vi "[SubVI]PMC.vi"(4 "Weight":dbl format="%#_13g", 6 "Speed":dbl format="%#_13g", 7 "Right Stride":bool, 9 "Offset  array":sgl[](array[numeric]), 10 "Max torque in":sgl=4.5, 11 "Left Stride":bool) -> (0 "output array":sgl[](array[numeric]), 1 "PMC Output":sgl[](array[numeric]), 3 "Set Point":dbl[](array[numeric]))   [LabVIEW 2018]
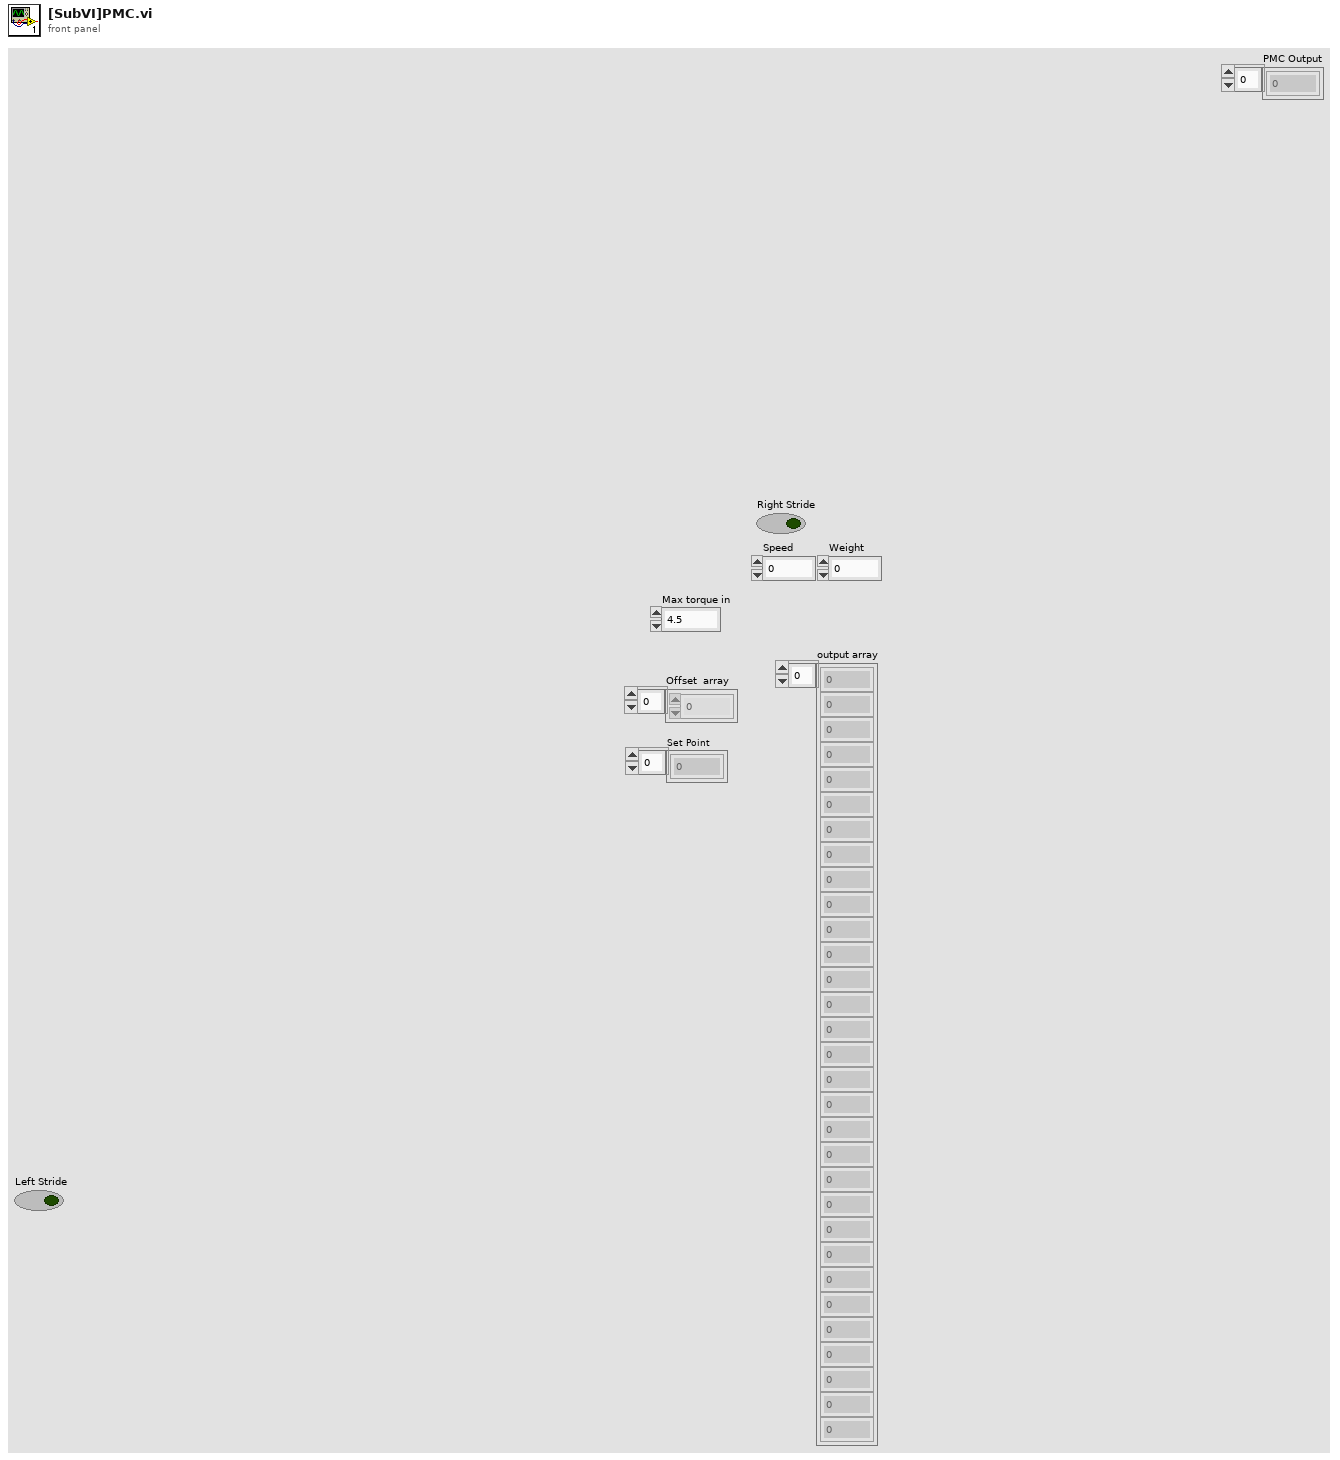
[diagram p1: front panel]
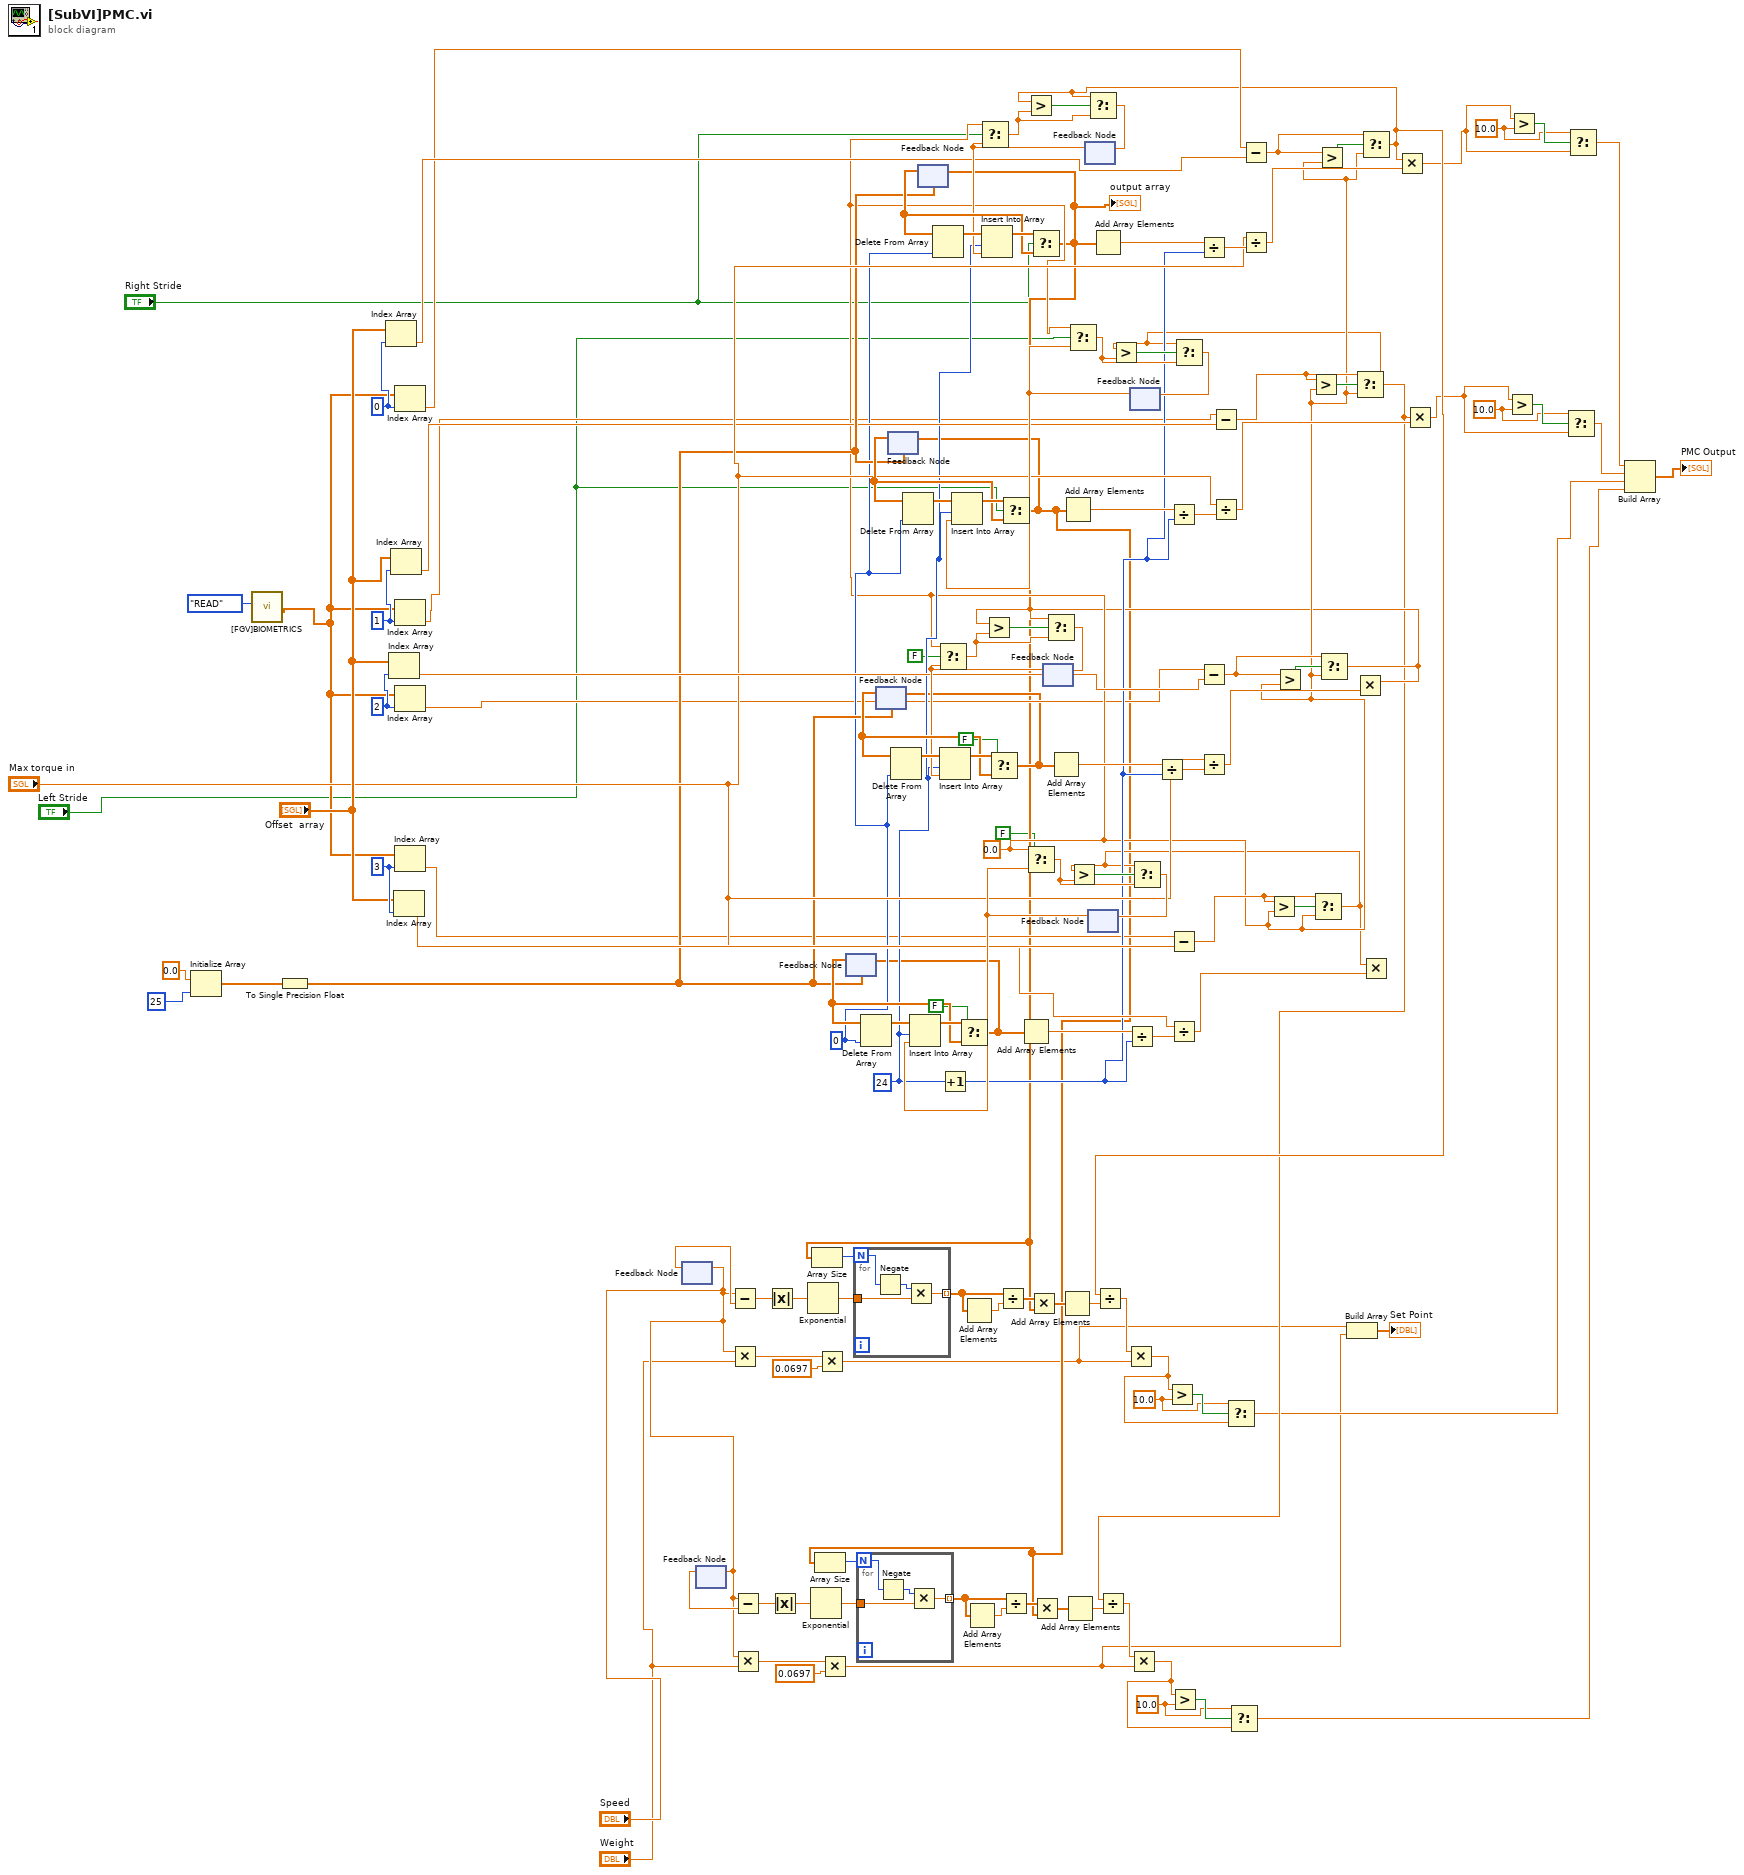
[diagram p0: block diagram]
diagram:
  w15 = 10.0 ("y")
  w19 = 10.0 ("y")
  w29 = 10.0 ("y")
  w44 = 10.0 ("y")
  w72 = u8 24 ("index")
  w70 = u8 0 ("index")
  w69 = sgl 0.0 ("t")
  w132 = 1 ("index")
  w130 = 0 ("index")
  w134 = 3 ("index")
  w133 = 2 ("index")
  n1 = Initialize Array(0.0 ("element"), 25 ("dimension size")) -> (w127:dbl[])
  n2 = call "[FGV]BIOMETRICS.vi"("Select"=enum16{"READ", "WRITE"}."READ") -> ("Data out"=w62:sgl[])  [unwired: 10 in]
  n3 = To Single Precision Float(number=w127) -> (single precision float=w75:sgl[])
  n4 = Index Array(array="Offset  array", index=w130) -> (element=w74:sgl)
  n5 = Index Array(array="Offset  array", index=w133) -> (element=w102:sgl)
  n6 = Index Array(array="Offset  array", index=w132) -> (element=w73:sgl)
  n7 = Index Array(array="Offset  array", index=w134) -> (element=w101:sgl)
  n8 = Index Array(array=w62, index=w130) -> (element=w66:sgl)
  n9 = Index Array(array=w62, index=w132) -> (element=w65:sgl)
  n10 = Index Array(array=w62, index=w133) -> (element=w68:sgl)
  n11 = Index Array(array=w62, index=w134) -> (element=w67:sgl)
  n12 = feedback #1() -> (w57:dbl)  [unwired: 1 in]
  n13 = feedback-in #1("Speed") -> ()
  n14 = feedback #2() -> (w26:dbl)  [unwired: 1 in]
  n15 = feedback-in #2("Speed") -> ()
  n16 = Subtract(x="Speed", y=w57) -> (x-y=w56:dbl)
  n17 = Multiply(x="Speed", y="Weight") -> (x*y=w48:dbl)
  n18 = Subtract(x="Speed", y=w26) -> (x-y=w41:dbl)
  n19 = Multiply(x="Speed", y="Weight") -> (x*y=w33:dbl)
  n20 = Absolute Value(x=w56) -> (abs(x)=w55:dbl)
  n21 = Absolute Value(x=w41) -> (abs(x)=w40:dbl)
  n22 = Exponential(1:w55) -> (0:w53:dbl)
  n23 = Exponential(1:w40) -> (0:w38:dbl)
  n24 = Multiply(x=w48, y=0.0697) -> (x*y=w7:dbl)
  n25 = Multiply(x=w33, y=0.0697) -> (x*y=w6:dbl)
  n26 = feedback #3(w75) -> (w109:sgl[])
  n27 = Delete From Array(array=w109, index=w70) -> (array with subset deleted=w111:sgl[])  [unwired: 1 in, 1 out]
  n28 = feedback #4(w75) -> (w118:sgl[])
  n29 = feedback #5(w75) -> (w83:sgl[])
  n30 = Delete From Array(array=w118, index=w70) -> (array with subset deleted=w120:sgl[])  [unwired: 1 in, 1 out]
  n31 = Delete From Array(array=w83, index=w70) -> (array with subset deleted=w85:sgl[])  [unwired: 1 in, 1 out]
  n32 = feedback #6(w75) -> (w92:sgl[])
  n33 = Delete From Array(array=w92, index=w70) -> (array with subset deleted=w94:sgl[])  [unwired: 1 in, 1 out]
  n34 = Increment(x=w72) -> (x+1=w71:u8)
  n35 = feedback #7() -> (w107:sgl)  [unwired: 1 in]
  n36 = Select(t=w69, s=FALSE, f=w107) -> (s? t:f=w124:sgl)
  n37 = Insert Into Array(array=w120, index=w72, new element=w107) -> (w121:sgl[])
  n38 = Select(t=w121, s=FALSE, f=w118) -> (s? t:f=w60:sgl[])
  n39 = feedback-in #4(w60) -> ()
  n40 = Add Array Elements(numeric array=w60) -> (sum=w122:sgl)
  n41 = feedback #8() -> (w81:sgl)  [unwired: 1 in]
  n42 = Select(t=w69, s="Right Stride", f=w81) -> (s? t:f=w98:sgl)
  n43 = Insert Into Array(array=w94, index=w72, new element=w81) -> (w95:sgl[])
  n44 = Select(t=w95, s="Right Stride", f=w92) -> (s? t:f=w12:sgl[])
  "output array" <- w12
  n45 = Array Size(array=w12) -> (size(s)=w54:i32)
  n46 = for {
    N: w54 -> [w136]
    tunnel: w53 -> [w137]
    tunnel: [w135] -> w52 mode=indexing
    n47 = Negate(x=w136) -> (-x=w138:i32)
    n48 = Multiply(x=w138, y=w137) -> (x*y=w135:dbl)
  }
  n49 = feedback-in #6(w12) -> ()
  n50 = Add Array Elements(numeric array=w52) -> (sum=w51:dbl)
  n51 = Divide(x=w52, y=w51) -> (x/y=w50:dbl[])
  n52 = Multiply(x=w50, y=w12) -> (x*y=w49:dbl[])
  n53 = Add Array Elements(numeric array=w49) -> (sum=w42:dbl)
  n54 = feedback #9() -> (w108:sgl)  [unwired: 1 in]
  n55 = Insert Into Array(array=w111, index=w72, new element=w108) -> (w112:sgl[])
  n56 = Select(t=w112, s=FALSE, f=w109) -> (s? t:f=w59:sgl[])
  n57 = feedback-in #3(w59) -> ()
  n58 = Add Array Elements(numeric array=w59) -> (sum=w113:sgl)
  n59 = Select(t=w69, s=FALSE, f=w108) -> (s? t:f=w115:sgl)
  n60 = Add Array Elements(numeric array=w12) -> (sum=w96:sgl)
  n61 = Divide(x=w113, y=w71) -> (x/y=w114:sgl)
  n62 = feedback #10() -> (w82:sgl)  [unwired: 1 in]
  n63 = Insert Into Array(array=w85, index=w72, new element=w82) -> (w86:sgl[])
  n64 = Select(t=w86, s="Left Stride", f=w83) -> (s? t:f=w21:sgl[])
  n65 = Array Size(array=w21) -> (size(s)=w39:i32)
  n66 = for {
    N: w39 -> [w140]
    tunnel: w38 -> [w141]
    tunnel: [w139] -> w37 mode=indexing
    n67 = Negate(x=w140) -> (-x=w142:i32)
    n68 = Multiply(x=w142, y=w141) -> (x*y=w139:dbl)
  }
  n69 = feedback-in #5(w21) -> ()
  n70 = Add Array Elements(numeric array=w37) -> (sum=w36:dbl)
  n71 = Divide(x=w37, y=w36) -> (x/y=w35:dbl[])
  n72 = Multiply(x=w35, y=w21) -> (x*y=w34:dbl[])
  n73 = Add Array Elements(numeric array=w21) -> (sum=w87:sgl)
  n74 = Add Array Elements(numeric array=w34) -> (sum=w27:dbl)
  n75 = Select(t=w69, s="Left Stride", f=w82) -> (s? t:f=w89:sgl)
  n76 = Divide(x=w122, y=w71) -> (x/y=w123:sgl)
  n77 = Divide(x=w87, y=w71) -> (x/y=w88:sgl)
  n78 = Subtract(x=w67, y=w101) -> (x-y=w103:sgl)
  n79 = Divide(x="Max torque in", y=w114) -> (x/y=w117:sgl)
  n80 = Divide(x=w96, y=w71) -> (x/y=w97:sgl)
  n81 = Subtract(x=w68, y=w102) -> (x-y=w105:sgl)
  n82 = Divide(x="Max torque in", y=w123) -> (x/y=w126:sgl)
  n83 = Subtract(x=w65, y=w73) -> (x-y=w77:sgl)
  n84 = Divide(x="Max torque in", y=w88) -> (x/y=w91:sgl)
  n85 = Subtract(x=w66, y=w74) -> (x-y=w79:sgl)
  n86 = Divide(x="Max torque in", y=w97) -> (x/y=w100:sgl)
  n87 = Greater?(x=w103, y=w69) -> (0:w104:bool)
  n88 = Greater?(x=w105, y=w69) -> (0:w106:bool)
  n89 = Greater?(x=w77, y=w69) -> (0:w78:bool)
  n90 = Select(t=w103, s=w104, f=w69) -> (s? t:f=w58:sgl)
  n91 = Greater?(x=w58, y=w115) -> (0:w110:bool)
  n92 = Select(t=w58, s=w110, f=w115) -> (s? t:f=w116:sgl)
  n93 = feedback-in #9(w116) -> ()
  n94 = Greater?(x=w79, y=w69) -> (0:w80:bool)
  n95 = Select(t=w105, s=w106, f=w69) -> (s? t:f=w64:sgl)
  n96 = Greater?(x=w64, y=w124) -> (0:w119:bool)
  n97 = Select(t=w64, s=w119, f=w124) -> (s? t:f=w125:sgl)
  n98 = feedback-in #7(w125) -> ()
  n99 = Build Array(w7, w6) -> (→"Set Point":dbl[])
  n100 = Select(t=w77, s=w78, f=w69) -> (s? t:f=w22:sgl)
  n101 = Divide(x=w22, y=w27) -> (x/y=w31:dbl)
  n102 = Greater?(x=w22, y=w89) -> (0:w84:bool)
  n103 = Multiply(x=w31, y=w6) -> (x*y=w28:dbl)
  n104 = Greater?(x=w28, y=w29) -> (0:w30:bool)
  n105 = Select(t=w22, s=w84, f=w89) -> (s? t:f=w90:sgl)
  n106 = feedback-in #10(w90) -> ()
  n107 = Select(t=w29, s=w30, f=w28) -> (s? t:f=w8:dbl)
  n108 = Multiply(x=w64, y=w126) -> ()  [unwired: 1 out]
  n109 = Select(t=w79, s=w80, f=w69) -> (s? t:f=w23:sgl)
  n110 = Greater?(x=w23, y=w98) -> (0:w93:bool)
  n111 = Select(t=w23, s=w93, f=w98) -> (s? t:f=w99:sgl)
  n112 = feedback-in #8(w99) -> ()
  n113 = Divide(x=w23, y=w42) -> (x/y=w46:dbl)
  n114 = Multiply(x=w46, y=w7) -> (x*y=w43:dbl)
  n115 = Greater?(x=w43, y=w44) -> (0:w45:bool)
  n116 = Select(t=w44, s=w45, f=w43) -> (s? t:f=w9:dbl)
  n117 = Multiply(x=w58, y=w117) -> ()  [unwired: 1 out]
  n118 = Multiply(x=w23, y=w100) -> (x*y=w18:sgl)
  n119 = Multiply(x=w22, y=w91) -> (x*y=w14:sgl)
  n120 = Greater?(x=w14, y=w15) -> (0:w16:bool)
  n121 = Greater?(x=w18, y=w19) -> (0:w20:bool)
  n122 = Select(t=w15, s=w16, f=w14) -> (s? t:f=w13:dbl)
  n123 = Select(t=w19, s=w20, f=w18) -> (s? t:f=w17:dbl)
  n124 = Build Array(w17, w13, w9, w8) -> (→"PMC Output":dbl[])
